vi "Dashboard Main.vi"() -> ()   [LabVIEW 2016]
uses:
  <vilib>/Utility/miscctls.llb/LVRowAndColumnTypeDef.ctl
  <vilib>/event_ctls.llb/eventvkey.ctl
  <vilib>/Rock Robotics/Network Tables/NT Read Numeric Array.vi
  <vilib>/Rock Robotics/Network Tables/NT Write Numeric Array.vi
  <vilib>/Rock Robotics/WPI/Dashboard/WPI_DashboardLogging Global.vi
panel:
  in  "Camera Settings Right":T1={"Frame Rate"=30, "Compression"=30, "Size"=1, "DB Camera Config"=FALSE} {"Frame Rate" scale=1.0..30.0; "Compression" scale=100.0..-1.0; "Size" items=["640x480", "320x240", "160x120"]}
  in  "Camera Name Right":string(combo)="No Camera Selection"
  out "Camera Info":cluster{"Mbps LED":bool, "Mbps":dbl, "fps":dbl} {"fps" format="%#.1g"; "Mbps" format="%#.1g"}
  in  "Camera Settings":T1={"Frame Rate"=30, "Compression"=30, "Size"=1, "DB Camera Config"=FALSE} {"Frame Rate" scale=1.0..30.0; "Compression" scale=100.0..-1.0; "Size" items=["640x480", "320x240", "160x120"]}
  in  "TCP":refnum<k5>
  in  "Rec Mode":enum32{"Stop", "Record", "Playback"}(radio)
  out "Robot IP":string
  out "Image Message":string="Timeout in Camera Communications"
  in  "Dashboard Tab":T2(tab)
  in  "Select Auto":string(combo)="Select Autonomous ..."
  out "NT Connection":bool
  out "MotorChart R":cluster{"Numeric":dbl, "Numeric":dbl}(graph)
  out "MotorChart L":cluster{"Numeric":dbl, "Numeric":dbl}(graph)
  out "MotorSliders R":cluster{"MotorSlide1":dbl, "MotorSlide2":dbl} {"MotorSlide2" scale=-1.0..1.0 scale format="%#_2e"; "MotorSlide1" scale=-1.0..1.0 scale format="%#_2e"}
  out "MotorSliders L":cluster{"MotorSlide1":dbl, "MotorSlide2":dbl} {"MotorSlide2" scale=-1.0..1.0 scale format="%#_2e"; "MotorSlide1" scale=-1.0..1.0 scale format="%#_2e"}
  out "Gyro":dbl(knob) scale=0.0..360.0
  out "JS1 Z":dbl(slide) scale=-1.0..1.0 scale format="%#_2e"
  out "JS1 Graph":cluster{"X":dbl, "Y":dbl}[](graph)
  out "JS1 Buttons":T3
  out "JS2 Z":dbl(slide) scale=-1.0..1.0 scale format="%#_2e"
  out "JS2 Graph":cluster{"X":dbl, "Y":dbl}[](graph)
  out "JS2 Buttons":T3
  out "Mode":T4(ring)=enum."Auto Disabled"
  out "Camera Image Right":T5(plugin-control)
  out "Left Encoder":dbl
  out "Right Encoder":dbl
  in  "Function Tuning":enum32{"Drive with PID", "Drive by Angle"}(tab)
  in  "Accel Distance":dbl=64.0
  in  "Min Speed":dbl=0.35
  in  "Drive P/I/D":dbl[](array[numeric])=[1.0, 0.0, 0.01]
  in  "Max Speed":dbl=0.6
  in  "Turn Speed":dbl=0.65
  in  "Linearity":dbl=0.6
  in  "Turn P/I/D":dbl[](array[numeric])=[0.25, 0.001, 0.0]
  in  "Autonomous Distances":T6(tab)
  in  "Station 1":dbl[](array[numeric])=[97.0, 30.0, -30.0, 120.0]
  in  "Station 2":dbl[](array[numeric])=[82.0, -48.0, 48.0, 120.0]
  in  "Station 3":dbl[](array[numeric])=[96.0, 30.0, -30.0, 120.0]
  in  "Drive Forward":dbl[](array[numeric])=[82.0, 0.0, 0.0, 0.0]
  in  "Gear and B":dbl[](array[numeric])=[82.0, -48.0, 0.0, 0.0]
  in  "Test Slider":dbl(slide) scale=0.0..100.0 scale format="%#_3g"
  in  "On/Off":bool caption="Solenoid"
  in  "Test Name":u16(ring) items=["Select the test to run..."]
  in  "Test Tree":string(tree)
  in  "Motor":cluster{"Value":dbl, "Enable":bool} {"Value" scale=-1.0..1.0 scale format="%#_3g"}
  out "Progress":T7 {"Test Progress" scale=0.0..100.0}
  in  "Rev/Fwd":cluster{"Forward":bool, "Reverse":bool}
  in  "Test Ring":u16(ring) items=["Monochrome", "Color"]
  out "Cmd Status":string
  in  "Execute Command":bool
  in  "Command Params":string[][](table)
  in  "Command Selection":i32(listbox)
  in  "CheckList":i32(listbox)
  out "Tree":string(tree)
  out "Camera Image":T5(plugin-control)
  in  "Camera Name":string(combo)="No Camera Selection"
  in  "Background":bool
  # "HW"
  # "HW"
  # "Joysticks"
  # "Drive Motors"
  # "Front"
  # "Right"
  # "Left"
  # "Back"
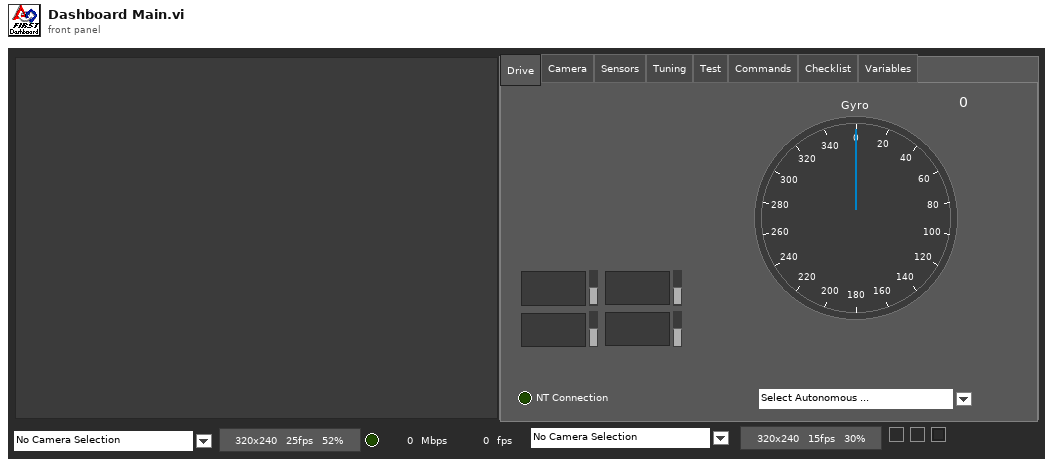
[diagram p1: front panel]
types:
  T1 = cluster{"Frame Rate":i32, "Compression":i32, "Size":u16, "DB Camera Config":bool}
  T2 = enum32{"Drive", "Camera", "Sensors", "Tuning", "Test", "Commands", "Checklist", "Variables"}
  T3 = cluster{bool, bool, bool, bool, bool, bool, bool, bool, bool, bool, bool, bool}
  T4 = enum8{"Tele-Op Disabled", "Tele-Op Enabled", "Auto Disabled", "Auto Enabled", "Test Disabled", "Test Enabled", "Disconnected", "No Code", "E-Stop"}
  T5 = typedef "IMAQ Image.ctl" = refnum<image>
  T6 = enum32{"Station 1", "Station 2", "Station 3", "Drive Forward", "Gear and Back"}
  T7 = cluster{"Test Progress":u8, "Test Progress Text":string}
  T8 = typedef "Image Type" = u32
  T9 = cluster{"IDs":cluster{"RPC field ID":u16, "Unique ID":u16}, "String":string}
  T10 = enum32{"Drive", "Basic", "Custom", "Test", "Checklist", "Variables"}
  T11 = cluster{"Error Strings":string, "Disable Counts":cluster{u16, u16}, "Rail Faults":cluster{u16, u16, u16}, "Robot IP":string, "DB Mode":u8, "Event Info":cluster{"Name":string, "Type":u8, "Number":u16, "Replay":u8}}
  T12 = cluster{"Storage":cluster{"Disk Free":u64, "RAM Block":u32, "RAM free":u32}, "CPU Utilization":cluster{"CPU % ISR":sgl, "CPU % Time Crit":sgl, "CPU % Timed Str":sgl, "CPU % High":sgl, "CPU % Above":sgl, "CPU % Normal":sgl, "CPU % Low":sgl}, "CAN":cluster{"% Bus Utilization":sgl, "Bus Off Cnt":u32, "TX_FIFO Full Cnt":u32, "Receive Error Cnt":u8, "Transmit Error Cnt":u8}, "HID":cluster{"HID Outputs":u32, "Rumble Low":u16, "Rumble High":u16}[]}
  T13 = cluster{"Status bits":cluster{"Test Mode":bool, "Autonomous":bool, "Enabled":bool, "Code Start":bool, "Brownout":bool, "Reserved 2":bool, "Reserved 3":bool, "E-Stop":bool}, "Code Trace":cluster{"Disabled":bool, "TeleOp":bool, "Auto":bool, "Test":bool}, "Controller Type":enum16{"unknown", "cRIO", "roboRio"}, "Code?":enum16{"unknown", "noCode", "code"}, "Battery V":dbl}
  T14 = cluster{"Control Bits":cluster{"TestMode":bool, "Autonomous":bool, "Enabled":bool, "FMS Present":bool, bool, bool, bool, "E-Stop":bool}, "Team Station ":u8, "Countdown":sgl, "Joystick Values":cluster{"Axes":dbl[], "Buttons":bool[], "POVs":i16[]}[]}
  T15 = cluster{"Axes":dbl[], "Buttons":bool[], "POVs":i16[]}[]
  T16 = cluster{"Axes":dbl[], "Buttons":bool[], "POVs":i16[]}
  T17 = cluster{"Buttons[0]":bool, "Buttons[1]":bool, "Buttons[2]":bool, "Buttons[3]":bool, "Buttons[4]":bool, "Buttons[5]":bool, "Buttons[6]":bool, "Buttons[7]":bool, "Buttons[8]":bool, "Buttons[9]":bool, "Buttons[10]":bool, "Buttons[11]":bool}
  T18 = cluster{"Camera Image":refnum<vi>, "Dashboard Tab":refnum<vi>, "Background":refnum<vi>, "Rec Mode":refnum<vi>, "Test Slider":refnum<vi>, "On/Off ":refnum<vi>, "Test Ring":refnum<vi>, "Rev/Fwd":refnum<vi>, "Test Name":refnum<vi>, "Motor":refnum<vi>, "Progress":refnum<vi>, "CheckList":refnum<vi>, "Tree":refnum<vi>, "Test Tree":refnum<vi>, "Command Params":refnum<vi>, "Command Selection":refnum<vi>, "Execute Command":refnum<vi>, "Cmd Status":refnum<vi>, "Camera Settings":refnum<vi>, "Camera Name":refnum<vi>, "Camera Info":refnum<vi>, "Camera Settings Right":refnum<vi>, "Camera Name Right":refnum<vi>, "Camera Image Right":refnum<vi>}
  T19 = cluster{"Operation":enum16{"Update", "Clear"}, "Color Box":u32}[]
  T20 = typedef "eventvkey.ctl" = enum16{"ASCII", "Enter", "Return", "Shift", "Ctrl", "Alt", "Cmd", "Opt", "Caps", "NumLock", "Clear", "Break", "Up", "Down", "Left", "Right", "Insert", "Delete", "Home", "End", "PageUp", "PageDown", "Escape", "Help", "Pause", "ScrollLock", "F1", "F2", "F3", "F4", "F5", "F6", "F7", "F8", "F9", "F10", "F11", "F12", "F13", "F14", "F15", "F16", "F17", "F18", "F19", "F20", "F21", "F22", "F23", "F24", "Play", "VolumeUp", "VolumeDown", "Mute", "Two Byte Char"}
  T21 = cluster{"Image Size":bool, "Image Type":bool, "Pixel Value":bool, "ROI Information":bool, "Zoom Factor":bool}
  T22 = cluster{"Operation":enum16{"Update", "Clear"}, "Color Box":u32}
  T23 = typedef "LVRowAndColumnTypeDef.ctl" = cluster{"Row":i32, "Column":i32}
  T24 = cluster{"Shift":bool, "Ctrl":bool, "Alt":bool, "Cmd":bool, "Opt":bool}
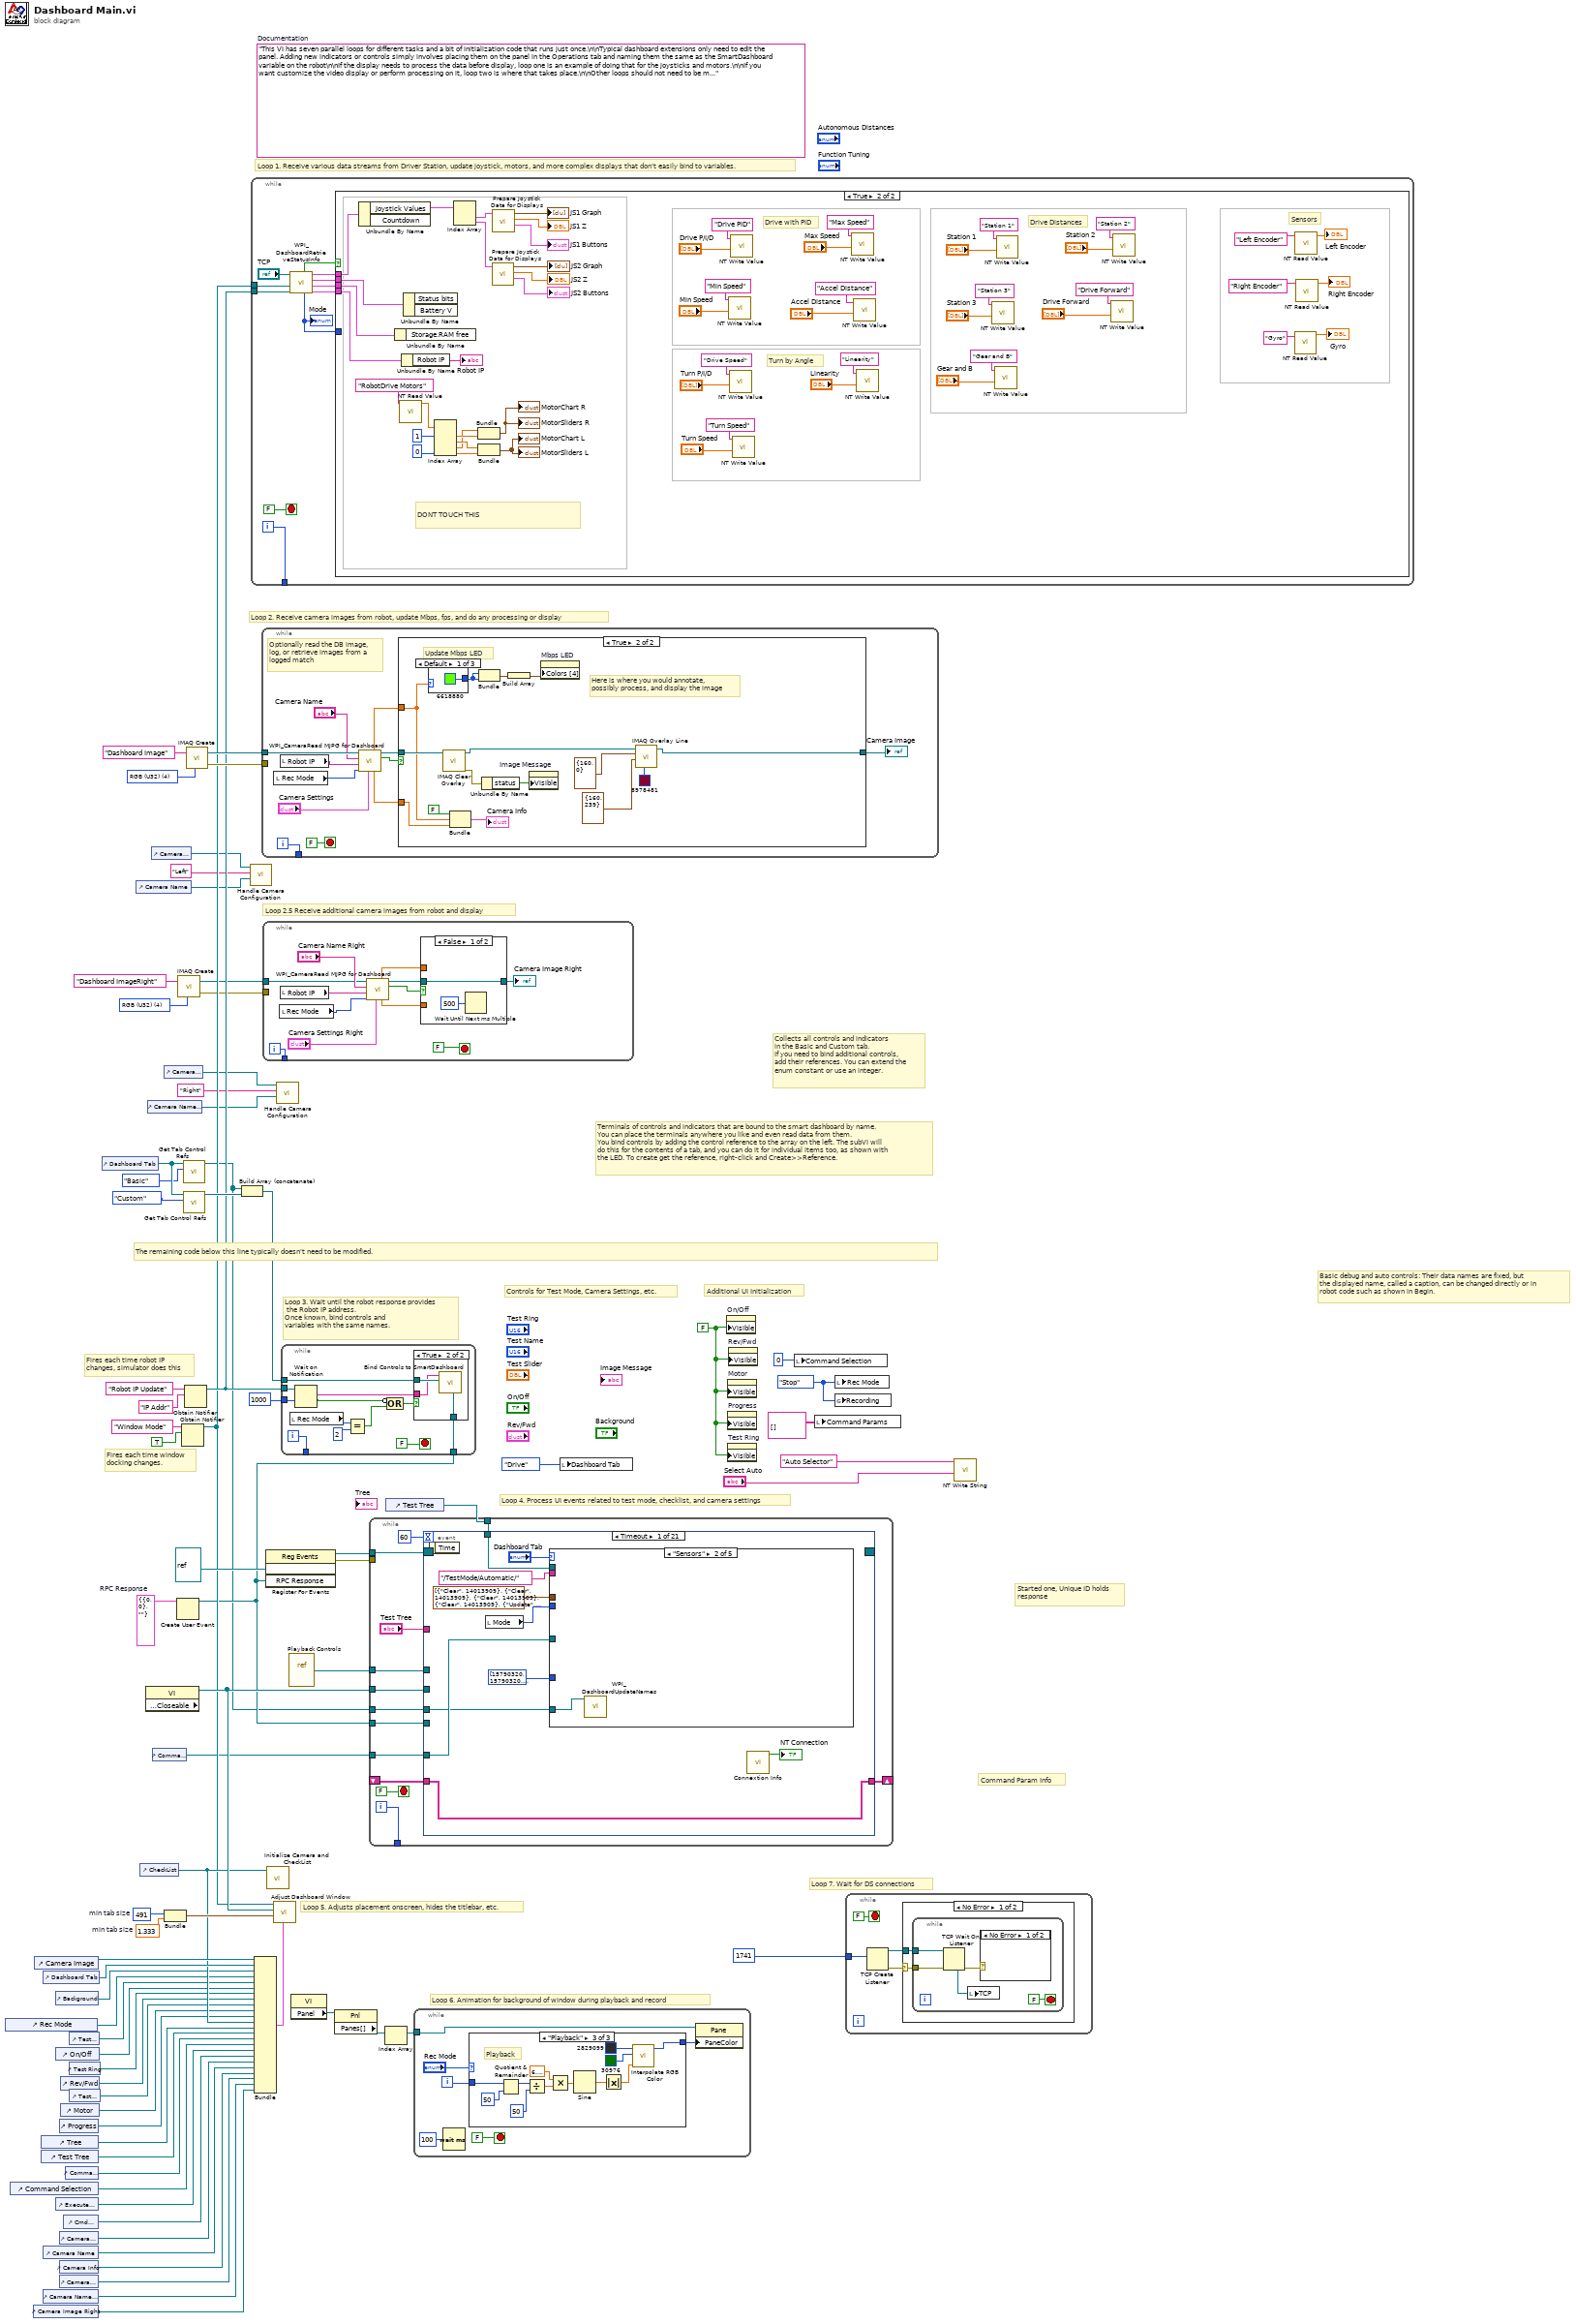
[diagram p0: block diagram]
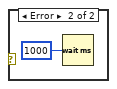
[diagram p3: hidden frame]
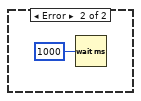
[diagram p4: hidden frame]
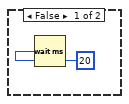
[diagram p5: hidden frame]
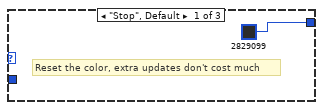
[diagram p6: hidden frame]
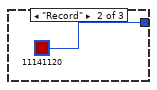
[diagram p7: hidden frame]
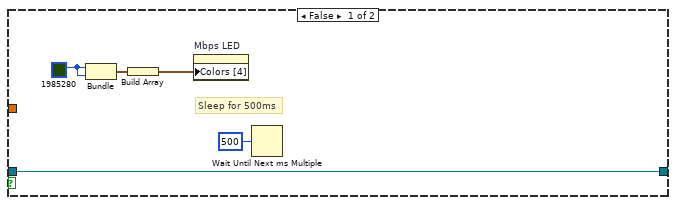
[diagram p9: hidden frame]
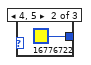
[diagram p10: hidden frame]
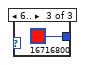
[diagram p11: hidden frame]
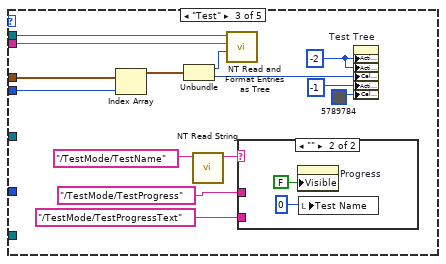
[diagram p13: hidden frame]
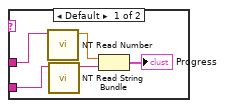
[diagram p14: hidden frame]
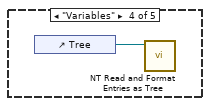
[diagram p15: hidden frame]
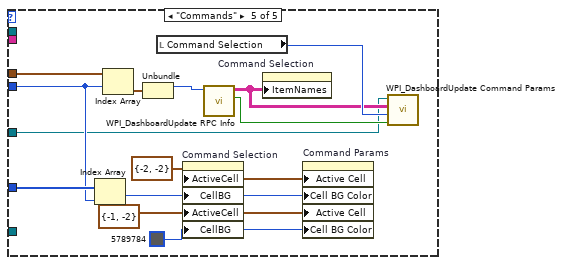
[diagram p16: hidden frame]
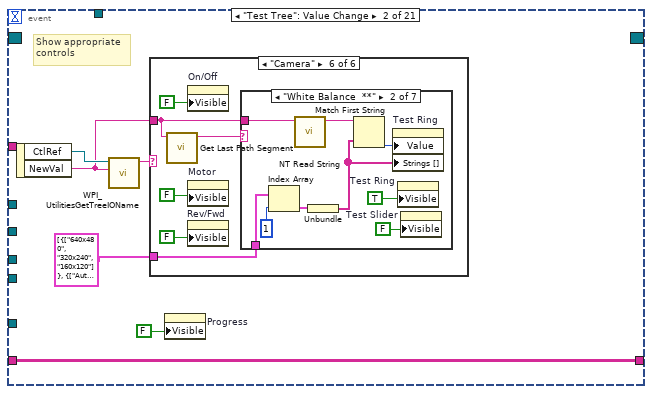
[diagram p17: hidden frame]
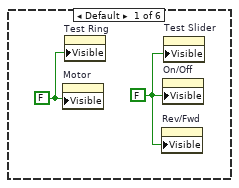
[diagram p18: hidden frame]
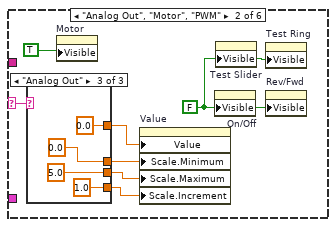
[diagram p19: hidden frame]
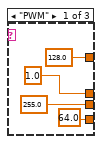
[diagram p20: hidden frame]
diagram:
  w11 = T8 4 items=["Grayscale (U8)", "Grayscale (I16)", "Grayscale (SGL)", "Complex (CSG)", "RGB (U32)", "HSL (U32)", "RGB (U64)"] ("Image Type")
  w27 = T9 {"IDs"={"RPC field ID"=0, "Unique ID"=0}, "String"=""}  # RPC Response
  w51 = 491  # min tab size
  w50 = 1.333  # min tab size
  w58 = enum32{"Stop", "Record", "Playback"}."Stop" ("Rec Mode")
  w34 = FALSE ("Visible")
  (unwired) "This VI has seven parallel loops for different tasks and a bit of initialization code that runs just once.\n\nTypical dashboard extensions only need to edit the panel. Adding new indicators or controls simply involves placing them on the panel in the Operations tab and naming them the same as the SmartDashboard variable on the robot\n\nIf the display needs to process the data before display, loop one is an example of doing that for the joysticks and motors.\n\nIf you want customize the video display or perform processing on it, loop two is where that takes place.\n\nOther loops should not need to be modified. They are pretty standard, and document the task they perform."  # Documentation
  w75 = T8 4 items=["Grayscale (U8)", "Grayscale (I16)", "Grayscale (SGL)", "Complex (CSG)", "RGB (U32)", "HSL (U32)", "RGB (U64)"] ("Image Type")
  # "Loop 2.5 Receive additional camera images from robot and display"
  # "Command Param Info"
  # "Started one, Unique ID holds\nresponse"
  # "Loop 7. Wait for DS connections"
  # "Basic debug and auto controls: Their data names are fixed, but\nthe displayed name, called a caption, can be changed directly or in\nrobot code such as shown in Begin."
  # "Controls for Test Mode, Camera Settings, etc."
  # "Additional UI Initialization"
  # "Loop 6. Animation for background of window during playback and record"
  # "Fires each time robot IP\nchanges, simulator does this"
  # "Fires each time window\ndocking changes."
  # "Collects all controls and indicators\nin the Basic and Custom tab.\nIf you need to bind additional controls,\nadd their references. You can extend the\nenum constant or use an integer."
  # "The remaining code below this line typically doesn't need to be modified."
  # "Loop 4. Process UI events related to test mode, checklist, and camera settings"
  # "Terminals of controls and indicators that are bound to the smart dashboard by name.\nYou can place the terminals anywhere you like and even read data from them.\nYou bind controls by adding the control reference to the array on the left. The subVI will\ndo this for the contents of a tab, and you can do it for individual items too, as shown with\nthe LED. To create get the reference, right-click and Create>>Reference."
  # "Loop 3. Wait until the robot response provides\n the Robot IP address.\nOnce known, bind controls and\nvariables with the same names."
  # "Loop 5. Adjusts placement onscreen, hides the titlebar, etc."
  # "Loop 1. Receive various data streams from Driver Station, update joystick, motors, and more complex displays that don't easily bind to variables."
  # "Loop 2. Receive camera images from robot, update Mbps, fps, and do any processing or display"
  n1 = control-ref of="Rec Mode"() -> (w40:refnum<vi>)
  n2 = control-ref of="Command Selection"() -> (w26:refnum<vi>)
  n3 = control-ref of="Camera Image Right"() -> (w2:refnum<vi>)
  n4 = control-ref of="Camera Image"() -> (w53:refnum<vi>)
  n5 = control-ref of="Tree"() -> (w44:refnum<vi>)
  n6 = control-ref of="Test Tree"() -> (w43:refnum<vi>)
  n7 = control-ref of="Dashboard Tab"() -> (w52:refnum<vi>)
  n8 = control-ref of="Camera Name"() -> (w17:refnum<vi>)
  n9 = control-ref of="Camera Name Right"() -> (w3:refnum<vi>)
  n10 = control-ref of="Background"() -> (w1:refnum<vi>)
  n11 = control-ref of="Execute Command"() -> (w28:refnum<vi>)
  n12 = control-ref of="On/Off"() -> (w38:refnum<vi>)
  n13 = control-ref of="Progress"() -> (w35:refnum<vi>)
  n14 = control-ref of="Camera Settings"() -> (w18:refnum<vi>)
  n15 = control-ref of="Camera Info"() -> (w16:refnum<vi>)
  n16 = control-ref of="Camera Settings Right"() -> (w4:refnum<vi>)
  n17 = control-ref of="Rev/Fwd"() -> (w36:refnum<vi>)
  n18 = control-ref of="Motor"() -> (w41:refnum<vi>)
  n19 = control-ref of="Cmd Status"() -> (w22:refnum<vi>)
  n20 = control-ref of="Command Params"() -> (w29:refnum<vi>)
  n21 = control-ref of="Test Slider"() -> (w39:refnum<vi>)
  n22 = control-ref of="Test Ring"() -> (w37:refnum<vi>)
  n23 = control-ref of="Test Name"() -> (w42:refnum<vi>)
  n24 = control-ref of="Dashboard Tab"() -> (w56:refnum<vi>)
  n25 = control-ref of="Camera Name"() -> (w19:refnum<vi>)
  n26 = control-ref of="CheckList"() -> (w45:refnum<vi>)
  n27 = property class="VI" props=["Front Panel.Closeable"]() -> (reference out=w57:refnum<vi>)  [unwired: 2 in, 2 out]
  n28 = control-ref of="Camera Name Right"() -> (w7:refnum<vi>)
  n29 = control-ref of="Camera Settings"() -> (w20:refnum<vi>)
  n30 = control-ref of="Command Params"() -> (w21:refnum<vi>)
  n31 = control-ref of="Camera Settings Right"() -> (w8:refnum<vi>)
  n32 = Bundle("min tab size"=w51, "min tab size"=w50) -> (w49:cluster{"min tab size":i32, "min tab size":dbl})  [unwired: 1 in]
  n33 = Create User Event(user event datatype=w27) -> (user event=w23:refnum<user-event>)  [unwired: 1 in, 1 out]
  n34 = call "IMAQ Create"("Image Name"="Dashboard ImageRight", "Image Type"=w11) -> ("New Image"=w10:T5, "error out"=w9:errorcluster)  [unwired: 2 in, 1 out]
  n35 = Obtain Notifier(name (unnamed)="Window Mode", notification data type=TRUE) -> (notifier out=w32:refnum<notifier>)  [unwired: 2 in, 2 out]
  n36 = call <vilib>:"Get Tab Control Refs.vi"("Page Index"=T10."Basic" ("Dashboard Tab"), "TabControl in"=w56) -> ("ControlsOnPage"=w15:refnum<vi>[])  [unwired: 9 in]
  n37 = call <vilib>:"Get Tab Control Refs.vi"("Page Index"=T10."Custom" ("Dashboard Tab"), "TabControl in"=w56) -> ("ControlsOnPage"=w55:refnum<vi>[])  [unwired: 9 in]
  n38 = Obtain Notifier(name (unnamed)="Robot IP Update", notification data type="IP Addr" ("name (unnamed)")) -> (notifier out=w33:refnum<notifier>)  [unwired: 2 in, 2 out]
  n39 = call "IMAQ Create"("Image Name"="Dashboard Image", "Image Type"=w75) -> ("New Image"=w73:T5, "error out"=w72:errorcluster)  [unwired: 2 in, 1 out]
  n40 = Build Array (concatenate)(w15, w55) -> (w54:refnum<vi>[])
  n41 = call "Handle Camera Configuration.vi"("CameraNameRef"=w19, "Camera File Name"="Left", "ClusterRef"=w20) -> ()  [unwired: 9 in]
  n42 = while {
    tunnel: [w85] -> _
    tunnel: w33 -> [w79]
    tunnel: w32 -> [w76]
    i -> [w85]
    stop <- FALSE stop-if-true
    n43 = call <vilib>:"WPI_DashboardRetrieveStatusInfo.vi"("Binding Refnum"=w79, "Window Mode Notifier"=w76, "TCP Cnx"="TCP") -> ("Power and Errors"=w80:T11, "Robot Metrics"=w83:T12, "Status Info"=w84:T13, "Control Info"=w81:T14, "Robot Mode"=w78:T4, "Process?"=w82:bool)  [unwired: 3 in]
    "Mode" <- w78
    n44 = case shown="True" w82 {
      tunnel: w84 -> [_ w141]
      tunnel: w83 -> [_ w140]
      tunnel: w81 -> [_ w139]
      tunnel: w80 -> [_ w138]
      tunnel: w78 -> [_ _]
      frame False {
        n45 = Wait (ms)(milliseconds to wait=u32 20) -> ()  [unwired: 1 out]
      }
      frame True {
        # "Sensors"
        # "Drive Distances"
        # "Turn by Angle"
        # "Drive with PID"
        # "DONT TOUCH THIS"
        n46 = Unbundle By Name(w139) -> ("Joystick Values"=w129:T15)  [unwired: 1 out]
        n47 = Unbundle By Name(w140) -> ()  [unwired: 1 out]
        n48 = call-poly <vilib>:"NT Read Value.vi"("Name"="RobotDrive Motors") -> ("Numeric Array"=w119:dbl[])  [unwired: 9 in, 1 out]
        n49 = Unbundle By Name(w138) -> ("Robot IP"=→"Robot IP":string)
        n50 = Unbundle By Name(w141) -> ()  [unwired: 2 out]
        n51 = Index Array(array=w119, index #1=1, index #4=0) -> (element #1=w133:dbl, element #2=w134:dbl, element #3=w132:dbl, element #4=w137:dbl)  [unwired: 2 in]
        n52 = Index Array(array=w129) -> (element #1=w128:T16, element #2=w124:T16)  [unwired: 2 in]
        n53 = Bundle("Numeric"=w132, "Numeric"=w133) -> (→"MotorChart R" →"MotorSliders R":cluster{"Numeric":dbl, "Numeric":dbl})  [unwired: 1 in]
        n54 = Bundle("Numeric"=w134, "Numeric"=w137) -> (→"MotorChart L" →"MotorSliders L":cluster{"Numeric":dbl, "Numeric":dbl})  [unwired: 1 in]
        n55 = call "Prepare Joystick Data for Displays.vi"("Joystick Values"=w124) -> ("Buttons"=→"JS2 Buttons":T17, "Z Axis"=→"JS2 Z":dbl, "Cartesian Data"=→"JS2 Graph":cluster{"X axis":dbl, "X axis":dbl}[])  [unwired: 8 in]
        n56 = call "Prepare Joystick Data for Displays.vi"("Joystick Values"=w128) -> ("Buttons"=→"JS1 Buttons":T17, "Z Axis"=→"JS1 Z":dbl, "Cartesian Data"=→"JS1 Graph":cluster{"X axis":dbl, "X axis":dbl}[])  [unwired: 8 in]
        n57 = call-poly <vilib>:"NT Write Value.vi"("Numeric"="Min Speed", "Name"="Min Speed") -> ()  [unwired: 9 in, 1 out]
        n58 = call-poly <vilib>:"NT Write Value.vi"("Numeric Array"="Turn P/I/D", "Name"="Drive Speed") -> ()  [unwired: 9 in, 1 out]
        n59 = call-poly <vilib>:"NT Write Value.vi"("Numeric Array"="Drive P/I/D", "Name"="Drive PID") -> ()  [unwired: 9 in, 1 out]
        n60 = call-poly <vilib>:"NT Write Value.vi"("Numeric"="Turn Speed", "Name"="Turn Speed") -> ()  [unwired: 9 in, 1 out]
        n61 = call-poly <vilib>:"NT Write Value.vi"("Numeric"="Max Speed", "Name"="Max Speed") -> ()  [unwired: 9 in, 1 out]
        n62 = call-poly <vilib>:"NT Write Value.vi"("Numeric"="Accel Distance", "Name"="Accel Distance") -> ()  [unwired: 9 in, 1 out]
        n63 = call-poly <vilib>:"NT Write Value.vi"("Numeric"="Linearity", "Name"="Linearity") -> ()  [unwired: 9 in, 1 out]
        n64 = call-poly <vilib>:"NT Write Value.vi"("Numeric Array"="Station 3", "Name"="Station 3") -> ()  [unwired: 9 in, 1 out]
        n65 = call-poly <vilib>:"NT Write Value.vi"("Numeric Array"="Gear and B", "Name"="Gear and B") -> ()  [unwired: 9 in, 1 out]
        n66 = call-poly <vilib>:"NT Write Value.vi"("Numeric Array"="Station 1", "Name"="Station 1") -> ()  [unwired: 9 in, 1 out]
        n67 = call-poly <vilib>:"NT Write Value.vi"("Numeric Array"="Drive Forward", "Name"="Drive Forward") -> ()  [unwired: 9 in, 1 out]
        n68 = call-poly <vilib>:"NT Write Value.vi"("Numeric Array"="Station 2", "Name"="Station 2") -> ()  [unwired: 9 in, 1 out]
        n69 = call-poly <vilib>:"NT Read Value.vi"("Name"="Gyro") -> ("Numeric"=→"Gyro":dbl)  [unwired: 9 in, 1 out]
        n70 = call-poly <vilib>:"NT Read Value.vi"("Name"="Left Encoder") -> ("Numeric"=→"Left Encoder":dbl)  [unwired: 9 in, 1 out]
        n71 = call-poly <vilib>:"NT Read Value.vi"("Name"="Right Encoder") -> ("Numeric"=→"Right Encoder":dbl)  [unwired: 9 in, 1 out]
      }
    }
  }
  n72 = Bundle("Camera Image"=w53, "Dashboard Tab"=w52, "Background"=w1, "Rec Mode"=w40, "Test Slider"=w39, "On/Off"=w38, "Test Ring"=w37, "Rev/Fwd"=w36, "Test Name"=w42, "Motor"=w41, "Progress"=w35, "CheckList"=w45, "Tree"=w44, "Test Tree"=w43, "Command Params"=w29, "Command Selection"=w26, "Execute Command"=w28, "Cmd Status"=w22, "Camera Settings"=w18, "Camera Name"=w17, "Camera Info"=w16, "Camera Settings Right"=w4, "Camera Name Right"=w3, "Camera Image Right"=w2) -> (w46:T18)  [unwired: 1 in]
  n73 = while {
    tunnel: w73 -> [w151]
    tunnel: w72 -> [_]
    tunnel: [w152] -> _
    i -> [w152]
    stop <- FALSE stop-if-true
    # "Optionally read the DB image,\nlog, or retrieve images from a\nlogged match"
    n74 = local read "Rec Mode"() -> (w147:enum32{"Stop", "Record", "Playback"})
    n75 = local read "Robot IP"() -> (w146:string)
    n76 = call <vilib>:"WPI_CameraRead MJPG for Dashboard.vi"("Camera Settings"="Camera Settings", "Rec Mode"=w147, "Robot IP"=w146, "Camera Name"="Camera Name", "Refnum in"=w151) -> ("Active"=w149:bool, "Refnum out"=w150:T5, "FPS"=w148:dbl, "Bandwidth (Mbps)"=w145:dbl)  [unwired: 3 in]
    n77 = case shown="True" w149 {
      tunnel: w150 -> [w154 w169]
      tunnel: w145 -> [_ w166]
      tunnel: w148 -> [_ w167]
      tunnel: [w154 w162] -> w142
      frame False {
        w156 = u32 1985280 ("Color Box")
        # "Sleep for 500ms"
        n78 = Bundle("Color Box"=w156, "Color Box"=w156) -> (w157:cluster{"Color Box":u32, "Color Box":u32})  [unwired: 1 out]
        n79 = Build Array(w157) -> (w155:cluster{"Color Box":u32, "Color Box":u32}[])
        n80 = property on="Mbps LED" class="Bool (strict)"("Colors [4]"=w155) -> ()  [unwired: 2 in, 2 out]
        n81 = Wait Until Next ms Multiple(millisecond multiple=u32 500) -> ()  [unwired: 1 out]
      }
      frame True {
        # "Here is where you would annotate,\npossibly process, and display the image"
        # "Update Mbps LED"
        n82 = case shown="Default" w166 {
          tunnel: [u32 6618880 ("Color Box") u32 16776722 ("Color Box") u32 16716800 ("Color Box")] -> w170
          frame Default {
          }
          frame 4, 5 {
          }
          frame 6.. {
          }
        }
        n83 = call "IMAQ Clear Overlay"("Image"=w169) -> ("error out"=w172:errorcluster, "Image Out"=w163:T5)  [unwired: 2 in, 7 out]
        n84 = Bundle(FALSE, "Bandwidth (Mbps)"=w166, "FPS"=w167) -> (→"Camera Info":cluster{bool, "Bandwidth (Mbps)":dbl, "FPS":dbl})  [unwired: 1 in]
        n85 = Bundle("Color Box"=w170, "Color Box"=w170) -> (w171:cluster{"Color Box":u32, "Color Box":u32})  [unwired: 1 out]
        n86 = Unbundle By Name(w172) -> ("status"=w173:bool)
        n87 = Build Array(w171) -> (w168:cluster{"Color Box":u32, "Color Box":u32}[])
        n88 = property on="Image Message" class="Str"("Visible"=w173) -> ()  [unwired: 2 in, 2 out]
        n89 = property on="Mbps LED" class="Bool (strict)"("Colors [4]"=w168) -> ()  [unwired: 2 in, 2 out]
        n90 = call "IMAQ Overlay Line"("Color"=u32 8978481, "End Point"=cluster{"X":i32, "Y":i32} {"X"=160, "Y"=239}, "Start Point"=cluster{"X":i32, "Y":i32} {"X"=160, "Y"=0}, "Image"=w163) -> ("Image Out"=w162:T5)  [unwired: 6 in, 1 out]
      }
    }
    "Camera Image" <- w142
  }
  n91 = while {
    tunnel: w10 -> [w187]
    tunnel: w9 -> [_]
    tunnel: [w181] -> _
    i -> [w181]
    stop <- FALSE stop-if-true
    n92 = local read "Rec Mode"() -> (w185:enum32{"Stop", "Record", "Playback"})
    n93 = local read "Robot IP"() -> (w186:string)
    n94 = call <vilib>:"WPI_CameraRead MJPG for Dashboard.vi"("Camera Settings"="Camera Settings Right", "Rec Mode"=w185, "Robot IP"=w186, "Camera Name"="Camera Name Right", "Refnum in"=w187) -> ("Active"=w180:bool, "Refnum out"=w183:T5, "FPS"=w178:dbl, "Bandwidth (Mbps)"=w179:dbl)  [unwired: 3 in]
    n95 = case shown="False" w180 {
      tunnel: w183 -> [w189 w191]
      tunnel: w179 -> [_ _]
      tunnel: w178 -> [_ _]
      tunnel: [w189 w191] -> w177
      frame False {
        n96 = Wait Until Next ms Multiple(millisecond multiple=u32 500) -> ()  [unwired: 1 out]
      }
      frame True {
      }
    }
    "Camera Image Right" <- w177
  }
  n97 = register-events(refnum<vi> refnum, w23) -> (reference out=w62:refnum<event-registration>, error out=w61:errorcluster)  [unwired: 2 in]
  n98 = call "Initialize Camera and CheckList.vi"("ListBox in"=w45) -> ()  [unwired: 11 in]
  n99 = call "Adjust Dashboard Window.vi"("Sizing Refnums"=w46, "Size Constraints"=w49, "VI"=w57, "WIn Mode"=w32) -> ()  [unwired: 8 in]
  n100 = call "Handle Camera Configuration.vi"("CameraNameRef"=w7, "Camera File Name"="Right", "ClusterRef"=w8) -> ()  [unwired: 9 in]
  n101 = while {
    tunnel: w54 -> [w203]
    tunnel: w33 -> [w201]
    tunnel: [w199] -> _
    tunnel: u32 1000 ("milliseconds to wait") -> [w198]
    tunnel: w23 -> [w192]
    i -> [w199]
    stop <- FALSE stop-if-true
    n102 = local read "Rec Mode"() -> (w194:enum32{"Stop", "Record", "Playback"})
    n103 = Wait on Notification(notifier=w201, timeout in ms (-1)=w198) -> (notification=w200:string, timed out?=w196:bool)  [unwired: 2 in, 2 out]
    n104 = Equal?(x=w194, y=u16 2 ("Rec Mode")) -> (x = y?=w195:bool)
    n105 = Compound Arithmetic op=OR(invert w196, w195) -> (w197:bool)
    n106 = case shown="True" w197 {
      tunnel: w203 -> [_ w206]
      tunnel: w200 -> [_ w205]
      tunnel: w192 -> [_ w204]
      frame False {
      }
      frame True {
        n107 = call <vilib>:"Bind Controls to SmartDashboard.vi"("RPC ref"=w204, "Bound Control Refs"=w206, "Server IP Address"=w205) -> ()  [unwired: 9 in]
      }
    }
  }
  n108 = vi-ref "Playback Controls.vi"() -> (w63:refnum<vi>)
  n109 = property class="VI"() -> ("Panel"=w65:refnum<vi>)  [unwired: 2 in, 2 out]
  n110 = property class="Pnl"(reference=w65) -> ("Panes[]"=w66:refnum<vi>[])  [unwired: 1 in, 2 out]
  n111 = Index Array(array=w66) -> (element=w64:refnum<vi>)  [unwired: 1 in]
  n112 = control-ref of="Test Tree"() -> (w67:refnum<vi>)
  n113 = while {
    tunnel: [w216] -> _
    tunnel: w67 -> [w215]
    tunnel: w63 -> [w214]
    tunnel: w62 -> [w213]
    tunnel: w61 -> [_]
    tunnel: w57 -> [w212]
    tunnel: w23 -> [w211]
    tunnel: w21 -> [w210]
    shift-right: [w209] -> _
    shift-left: _ -> [w208]
    tunnel: w15 -> [w207]
    i -> [w216]
    stop <- FALSE stop-if-true
    n114 = event shown="[0] Timeout" {
      selector: w213 -> [_ _ _ _ _ _ _ _ _ _ _ _ _ _ _ _ _ _ _ _ _]
      dyn-events: [_ _ _ _ _ _ _ _ _ _ _ _ _ _ _ _ w472 _ _ _ _] -> _
      timeout: u32 60 ("milliseconds to wait") -> [_ _ _ _ _ _ _ _ _ _ _ _ _ _ _ _ _ _ _ _ _]
      tunnel: w215 -> [w228 _ _ _ _ _ _ _ _ _ _ _ _ _ _ _ _ _ _ _ _]
      tunnel: "Test Tree" -> [_ _ _ _ _ _ _ _ _ _ _ w439 w447 w449 w453 w461 _ _ _ _ _]
      tunnel: w214 -> [_ _ _ _ _ _ _ _ _ _ _ _ _ _ _ _ w474 _ w492 _ _]
      tunnel: w212 -> [_ _ _ _ _ _ _ _ _ _ _ _ _ _ _ _ w470 _ _ _ _]
      tunnel: w211 -> [_ _ _ _ _ _ _ _ _ _ _ _ _ _ _ _ w466 _ _ _ _]
      tunnel: w210 -> [w223 _ _ _ _ _ w390 _ _ _ _ _ _ _ _ _ _ _ _ _ _]
      tunnel: [w222 w267 w369 w374 w383 w387 w388 w397 w407 w414 w426 w438 w445 w448 w452 w460 w465 w487 w489 w493 w504] -> w209
      tunnel: w208 -> [w222 w267 w369 w374 w383 w387 w388 _ _ w414 w426 w438 w445 w448 w452 w460 w465 w487 w489 w493 w504]
      tunnel: w207 -> [w220 _ _ _ _ _ _ _ _ _ _ _ _ _ _ _ _ _ _ _ _]
      event Timeout {
        n115 = event-data() -> ()  [unwired: 1 in, 1 out]
        n116 = local read "Mode"() -> (w225:T4)
        n117 = case shown="\"Sensors\"" "Dashboard Tab" {
          tunnel: w228 -> [_ _ w244 _ _]
          tunnel: "/TestMode/Automatic/" ("Name Pattern") -> [_ _ w243 _ _]
          tunnel: T19 [{"Operation"=enum."Clear", "Color Box"=14013909}, {"Operation"=enum."Clear", "Color Box"=14013909}, {"Operation"=enum."Clear", "Color Box"=14013909}, {"Operation"=enum."Clear", "Color Box"=14013909}, {"Operation"=enum."Update", "Color Box"=14013909}, {"Operation"=enum."Update", "Color Box"=16777215}, {"Operation"=enum."Clear", "Color Box"=14013909}, {"Operation"=enum."Clear", "Color Box"=14013909}, {"Operation"=enum."Clear", "Color Box"=14013909}] -> [_ _ w236 _ w260]
          tunnel: w225 -> [_ _ w235 _ w259]
          tunnel: u32[] [15790320, 15790320, 15790320, 15790320, 16777215, 16777215, 15790320, 15790320, 15790320] -> [_ _ _ _ w265]
          tunnel: w223 -> [_ _ _ _ w253]
          tunnel: w220 -> [_ w230 _ _ _]
          frame "Tuning", Default {
          }
          frame "Sensors" {
            n118 = call <vilib>:"WPI_DashboardUpdateNames.vi"("Controls on Tab"=w230) -> ()  [unwired: 11 in]
          }
          frame "Test" {
            w242 = -2 ("Active Item:Row Number")
            n119 = Index Array(array=w236, index=w235) -> (element=w237:T22)
            n120 = Unbundle(w237) -> ("Operation"=w238:enum16{"Update", "Clear"}, "Color Box"=w239:u32)
            n121 = call <vilib>:"NT Read String.vi"("Name"="/TestMode/TestName") -> ("String"=w233:string)  [unwired: 9 in, 1 out]
            n122 = call <vilib>:"NT Read and Format Entries as Tree.vi"("Operation"=w238, "Name Pattern"=w243, "Tree Refnum"=w244) -> ()  [unwired: 7 in, 2 out]
            n123 = case shown="\"\"" w233 {
              tunnel: "/TestMode/TestProgress" ("Name") -> [w246 _]
              tunnel: "/TestMode/TestProgressText" ("Name") -> [w245 _]
              frame Default {
                n124 = call <vilib>:"NT Read Number.vi"("Name"=w246) -> ("Numeric"=w247:dbl)  [unwired: 9 in, 1 out]
                n125 = call <vilib>:"NT Read String.vi"("Name"=w245) -> ("String"=w248:string)  [unwired: 9 in, 1 out]
                n126 = Bundle("Numeric"=w247, "String"=w248) -> (→"Progress":cluster{"Numeric":dbl, "String":string})  [unwired: 1 in]
              }
              frame "" {
                n127 = property on="Progress" class="Clust (strict)"("Visible"=FALSE) -> ()  [unwired: 2 in, 2 out]
                n128 = local write "Test Name"(u16 0) -> ()
              }
            }
            n129 = property on="Test Tree" class="Tree (strict)"("Active Item Row Number"=w242, "ActiveColNum"=w242, "CellBG"=w239, "Active Item Row Number"=-1 ("Active Item:Row Number"), "CellBG"=u32 5789784 ("Color Box")) -> ()  [unwired: 2 in, 2 out]
          }
          frame "Variables" {
            n130 = control-ref of="Tree"() -> (w252:refnum<vi>)
            n131 = call <vilib>:"NT Read and Format Entries as Tree.vi"("Tree Refnum"=w252) -> ()  [unwired: 9 in, 2 out]
          }
          frame "Commands" {
            w261 = u32 5789784 ("Color Box")
            w262 = T23 {"Row"=-1, "Column"=-2} ("Active Cell:Active Cell")
            w264 = T23 {"Row"=-2, "Column"=-2} ("Active Cell:Active Cell")
            n132 = Index Array(array=w265, index=w259) -> (element=w263:u32)
            n133 = Index Array(array=w260, index=w259) -> (element=w258:T22)
            n134 = Unbundle(w258) -> ("Operation"=w257:enum16{"Update", "Clear"})  [unwired: 1 out]
            n135 = local read "Command Selection"() -> (w256:i32)
            n136 = property on="Command Selection" class="MCListbox (strict)"("ActiveCell"=w264, "CellBG"=w263, "ActiveCell"=w262, "CellBG"=w261) -> ()  [unwired: 2 in, 2 out]
            n137 = call <vilib>:"WPI_DashboardUpdate RPC Info.vi"("Operation"=w257) -> ("update"=w255:bool, "commands"=w254:string[][])  [unwired: 9 in]
            n138 = property on="Command Selection" class="MCListbox (strict)"("ItemNames"=w254) -> ()  [unwired: 2 in, 2 out]
            n139 = property on="Command Params" class="Tbl (strict)"("Active Cell"=w264, "Cell BG Color"=w263, "Active Cell"=w262, "Cell BG Color"=w261) -> ()  [unwired: 2 in, 2 out]
            n140 = call <vilib>:"WPI_DashboardUpdate Command Params.vi"("Update"=w255, "NewVal"=w256, "Commands"=w254, "Param Tbl"=w253) -> ()  [unwired: 7 in, 1 out]
          }
        }
        n141 = call <vilib>:"Connextion Info.vi"() -> ("Connected"=→"NT Connection":bool)  [unwired: 10 in, 1 out]
      }
      event "Test Tree": Value Change {
        # "Show appropriate\ncontrols"
        n142 = event-data() -> ("CtlRef"=w270:refnum<vi>, "NewVal"=w268:string)  [unwired: 1 in]
        n143 = call <vilib>:"WPI_UtilitiesGetTreeIOName.vi"("NewVal"=w268, "TreeControl in"=w270) -> ("I/O Name"=w271:string)  [unwired: 9 in]
        n144 = case shown="\"Camera\"" w271 {
          selector: w271 -> [_ w278 _ w300 w309 _]
          tunnel: w268 -> [_ _ w297 w299 _ w316]
          tunnel: cluster{string[]}[] [{["640x480", "320x240", "160x120"]}, {["Auto", "Fixed indoor", "Fixed outdoor 1", "Fixed outdoor 2", "Fixed fluorescent 1", "Fixed fluorescent 2", "Hold current"]}, {["Auto", "Flicker-free 50 Hz", "Flicker-free 60 Hz", "Hold current"]}, {["None", "Prioritize frame rate", "Prioritize image quality"]}, {["Monochrome", "Color"]}] -> [_ _ _ _ _ w315]
          frame Default {
            w273 = FALSE ("Visible")
            w272 = FALSE ("Visible")
            n145 = property on="Motor" class="Clust (strict)"("Visible"=w272) -> ()  [unwired: 2 in, 2 out]
            n146 = property on="Test Ring" class="Ring (strict)"("Visible"=w272) -> ()  [unwired: 2 in, 2 out]
            n147 = property on="Rev/Fwd" class="Clust (strict)"("Visible"=w273) -> ()  [unwired: 2 in, 2 out]
            n148 = property on="On/Off" class="Bool (strict)"("Visible"=w273) -> ()  [unwired: 2 in, 2 out]
            n149 = property on="Test Slider" class="Slide (strict)"("Visible"=w273) -> ()  [unwired: 2 in, 2 out]
          }
          frame "Analog Out", "Motor", "PWM" {
            w279 = FALSE ("Visible")
            n150 = case shown="\"Analog Out\"" w278 {
              tunnel: [1.0 ("Value") -1.0 ("Value") 0.0 ("Value")] -> w277
              tunnel: [255.0 ("Value") 1.0 ("Value") 5.0 ("Value")] -> w276
              tunnel: [128.0 ("Value") 0.0 ("Value") 0.0 ("Value")] -> w275
              tunnel: [64.0 ("Value") 0.5 ("Value") 1.0 ("Value")] -> w274
              frame "PWM" {
              }
              frame "Motor", Default {
              }
              frame "Analog Out" {
              }
            }
            n151 = property on="Motor" class="Clust (strict)"("Visible"=TRUE) -> ()  [unwired: 2 in, 2 out]
            n152 = property on="Value" class="Slide (strict)"("Value"=w275, "Scale.Minimum"=w277, "Scale.Maximum"=w276, "Scale.Increment"=w274) -> ()  [unwired: 2 in, 2 out]
            n153 = property on="On/Off" class="Bool (strict)"("Visible"=w279) -> ()  [unwired: 2 in, 2 out]
            n154 = property on="Test Slider" class="Slide (strict)"("Visible"=w279) -> ()  [unwired: 2 in, 2 out]
            n155 = property on="Test Ring" class="Ring (strict)"("Visible"=w279) -> ()  [unwired: 2 in, 2 out]
            n156 = property on="Rev/Fwd" class="Clust (strict)"("Visible"=w279) -> ()  [unwired: 2 in, 2 out]
          }
          frame "Servo" {
            w295 = FALSE ("Visible")
            n157 = call <vilib>:"NT Read Number.vi"("Name"=w297) -> ("Numeric"=w296:dbl)  [unwired: 9 in, 1 out]
            n158 = property on="Test Slider" class="Slide (strict)"("Visible"=TRUE, "Scale.Maximum"=170.0 ("Scale.Range:Maximum")) -> ()  [unwired: 2 in, 2 out]
            n159 = local write "Test Slider"(w296) -> ()
            n160 = property on="Motor" class="Clust (strict)"("Visible"=w295) -> ()  [unwired: 2 in, 2 out]
            n161 = property on="Rev/Fwd" class="Clust (strict)"("Visible"=w295) -> ()  [unwired: 2 in, 2 out]
            n162 = property on="On/Off" class="Bool (strict)"("Visible"=w295) -> ()  [unwired: 2 in, 2 out]
            n163 = property on="Test Ring" class="Ring (strict)"("Visible"=w295) -> ()  [unwired: 2 in, 2 out]
          }
          frame "Relay", "Solenoid" {
            w298 = FALSE ("Visible")
            n164 = property on="Motor" class="Clust (strict)"("Visible"=w298) -> ()  [unwired: 2 in, 2 out]
            n165 = property on="Test Slider" class="Slide (strict)"("Visible"=w298) -> ()  [unwired: 2 in, 2 out]
            n166 = Search and Replace String(input string=w299, search string="/Value  **", replace string="/Direction") -> (result string=w305:string)  [unwired: 5 in, 3 out]
            n167 = property on="Test Ring" class="Ring (strict)"("Visible"=w298) -> ()  [unwired: 2 in, 2 out]
            n168 = call <vilib>:"NT Read String.vi"("Name"=w305) -> ("String"=w303:string)  [unwired: 9 in, 1 out]
            n169 = Equal?(x="Both directions", y=w303) -> (x = y?=w301:bool)
            n170 = Not(x=w301) -> (.not. x?=w302:bool)
            n171 = property on="Rev/Fwd" class="Clust (strict)"("Visible"=w301) -> ()  [unwired: 2 in, 2 out]
            n172 = property on="On/Off" class="Bool (strict)"("Visible"=w302, "Caption.Text"=w300) -> ()  [unwired: 2 in, 2 out]
          }
          frame "Compressor", "Digital Out" {
            w308 = FALSE ("Visible")
            # "Get direction and finish"
            n173 = property on="Motor" class="Clust (strict)"("Visible"=w308) -> ()  [unwired: 2 in, 2 out]
            n174 = property on="Test Slider" class="Slide (strict)"("Visible"=w308) -> ()  [unwired: 2 in, 2 out]
            n175 = property on="Test Ring" class="Ring (strict)"("Visible"=w308) -> ()  [unwired: 2 in, 2 out]
            n176 = property on="On/Off" class="Bool (strict)"("Visible"=TRUE, "Caption.Text"=w309) -> ()  [unwired: 2 in, 2 out]
            n177 = property on="Rev/Fwd" class="Clust (strict)"("Visible"=FALSE) -> ()  [unwired: 2 in, 2 out]
          }
          frame "Camera" {
            n178 = call <vilib>:"Get Last Path Segment.vi"("String in"=w316) -> ("String out"=w317:string)  [unwired: 10 in]
            n179 = property on="On/Off" class="Bool (strict)"("Visible"=FALSE) -> ()  [unwired: 2 in, 2 out]
            n180 = property on="Motor" class="Clust (strict)"("Visible"=FALSE) -> ()  [unwired: 2 in, 2 out]
            n181 = property on="Rev/Fwd" class="Clust (strict)"("Visible"=FALSE) -> ()  [unwired: 2 in, 2 out]
            n182 = case shown="\"White Balance  **\"" w317 {
              tunnel: w316 -> [w323 w332 w341 w350 w359 _ w365]
              tunnel: w315 -> [w321 w329 w338 w347 w356 _ _]
              frame "Size  **" {
                n183 = Index Array(array=w321) -> (element=w320:cluster{string[]})  [unwired: 1 in]
                n184 = call <vilib>:"NT Read String.vi"("Name"=w323) -> ("String"=w322:string)  [unwired: 9 in, 1 out]
                n185 = Unbundle(w320) -> (w318:string[])
                n186 = Match First String(2:w318, 3:w322) -> (0:w319:i32)  [unwired: 1 out]
                n187 = property on="Test Ring" class="Ring (strict)"("Value"=w319, "Strings []"=w318) -> ()  [unwired: 2 in, 2 out]
                n188 = property on="Test Ring" class="Ring (strict)"("Visible"=TRUE) -> ()  [unwired: 2 in, 2 out]
                n189 = property on="Test Slider" class="Slide (strict)"("Visible"=FALSE) -> ()  [unwired: 2 in, 2 out]
              }
              frame "White Balance  **" {
                n190 = Index Array(array=w329, index=1) -> (element=w330:cluster{string[]})
                n191 = call <vilib>:"NT Read String.vi"("Name"=w332) -> ("String"=w331:string)  [unwired: 9 in, 1 out]
                n192 = Unbundle(w330) -> (w327:string[])
                n193 = Match First String(2:w327, 3:w331) -> (0:w326:i32)  [unwired: 1 out]
                n194 = property on="Test Ring" class="Ring (strict)"("Value"=w326, "Strings []"=w327) -> ()  [unwired: 2 in, 2 out]
                n195 = property on="Test Ring" class="Ring (strict)"("Visible"=TRUE) -> ()  [unwired: 2 in, 2 out]
                n196 = property on="Test Slider" class="Slide (strict)"("Visible"=FALSE) -> ()  [unwired: 2 in, 2 out]
              }
              frame "Exposure  **" {
                n197 = Index Array(array=w338, index=2) -> (element=w339:cluster{string[]})
                n198 = call <vilib>:"NT Read String.vi"("Name"=w341) -> ("String"=w340:string)  [unwired: 9 in, 1 out]
                n199 = Unbundle(w339) -> (w335:string[])
                n200 = Match First String(2:w335, 3:w340) -> (0:w336:i32)  [unwired: 1 out]
                n201 = property on="Test Ring" class="Ring (strict)"("Value"=w336, "Strings []"=w335) -> ()  [unwired: 2 in, 2 out]
                n202 = property on="Test Ring" class="Ring (strict)"("Visible"=TRUE) -> ()  [unwired: 2 in, 2 out]
                n203 = property on="Test Slider" class="Slide (strict)"("Visible"=FALSE) -> ()  [unwired: 2 in, 2 out]
              }
              frame "Exposure Priority  **" {
                n204 = Index Array(array=w347, index=3) -> (element=w348:cluster{string[]})
                n205 = call <vilib>:"NT Read String.vi"("Name"=w350) -> ("String"=w349:string)  [unwired: 9 in, 1 out]
                n206 = Unbundle(w348) -> (w344:string[])
                n207 = Match First String(2:w344, 3:w349) -> (0:w345:i32)  [unwired: 1 out]
                n208 = property on="Test Ring" class="Ring (strict)"("Value"=w345, "Strings []"=w344) -> ()  [unwired: 2 in, 2 out]
                n209 = property on="Test Ring" class="Ring (strict)"("Visible"=TRUE) -> ()  [unwired: 2 in, 2 out]
                n210 = property on="Test Slider" class="Slide (strict)"("Visible"=FALSE) -> ()  [unwired: 2 in, 2 out]
              }
              frame "Color Enable  **" {
                n211 = Index Array(array=w356, index=4) -> (element=w357:cluster{string[]})
                n212 = call <vilib>:"NT Read String.vi"("Name"=w359) -> ("String"=w358:string)  [unwired: 9 in, 1 out]
                n213 = Unbundle(w357) -> (w353:string[])
                n214 = Match First String(2:w353, 3:w358) -> (0:w354:i32)  [unwired: 1 out]
                n215 = property on="Test Ring" class="Ring (strict)"("Value"=w354, "Strings []"=w353) -> ()  [unwired: 2 in, 2 out]
                n216 = property on="Test Ring" class="Ring (strict)"("Visible"=TRUE) -> ()  [unwired: 2 in, 2 out]
                n217 = property on="Test Slider" class="Slide (strict)"("Visible"=FALSE) -> ()  [unwired: 2 in, 2 out]
              }
              frame Default {
                n218 = property on="Test Ring" class="Ring (strict)"("Visible"=FALSE) -> ()  [unwired: 2 in, 2 out]
                n219 = property on="Test Slider" class="Slide (strict)"("Visible"=FALSE) -> ()  [unwired: 2 in, 2 out]
              }
              frame "Brightness  **", "Color Level  **", "Compression  **", "FPS  **", "Sharpness  **" {
                n220 = call <vilib>:"NT Read Number.vi"("Name"=w365) -> ("Numeric"=w364:dbl)  [unwired: 9 in, 1 out]
                n221 = local write "Test Slider"(w364) -> ()
                n222 = property on="Test Slider" class="Slide (strict)"("Visible"=TRUE, "Scale.Maximum"=100.0 ("Scale.Range:Maximum")) -> ()  [unwired: 2 in, 2 out]
                n223 = property on="Test Ring" class="Ring (strict)"("Visible"=FALSE) -> ()  [unwired: 2 in, 2 out]
              }
            }
          }
        }
        n224 = property on="Progress" class="Clust (strict)"("Visible"=FALSE) -> ()  [unwired: 2 in, 2 out]
      }
      event "Test Name": Mouse Enter {
        # "Populate the ring with the list of tests"
        n225 = event-data() -> ()  [unwired: 1 in, 1 out]
        n226 = call <vilib>:"NT Read String Array.vi"("Name"="/TestMode/TestList") -> ("String Array"=w373:string[])  [unwired: 9 in, 1 out]
        n227 = Build Array (concatenate)("Select the test to run...", w373) -> (w372:string[])
        n228 = property on="Test Name" class="Ring (strict)"("Strings []"=w372) -> ()  [unwired: 2 in, 2 out]
      }
      event "Test Name": Value Change {
        w375 = FALSE ("Visible")
        # "Tell the robot the test name to run"
        n229 = event-data() -> ("NewVal"=w379:u16)  [unwired: 1 in]
        n230 = property on="Test Name" class="Ring (strict)"() -> ("Strings []"=w380:string[])  [unwired: 2 in, 2 out]
        n231 = local write "Progress"(T7 {"Test Progress"=0, "Test Progress Text"=""} ("Progress")) -> ()
        n232 = Index Array(array=w380, index=w379) -> (element=w378:string)
        n233 = call <vilib>:"NT Write String.vi"("String"=w378, "Name"="/TestMode/TestName") -> ()  [unwired: 9 in, 1 out]
        n234 = property on="Progress" class="Clust (strict)"("Visible"=TRUE) -> ()  [unwired: 2 in, 2 out]
        n235 = property on="Motor" class="Clust (strict)"("Visible"=w375) -> ()  [unwired: 2 in, 2 out]
        n236 = property on="Test Slider" class="Slide (strict)"("Visible"=w375) -> ()  [unwired: 2 in, 2 out]
        n237 = property on="On/Off" class="Bool (strict)"("Visible"=w375) -> ()  [unwired: 2 in, 2 out]
        n238 = property on="Rev/Fwd" class="Clust (strict)"("Visible"=w375) -> ()  [unwired: 2 in, 2 out]
        n239 = property on="Test Ring" class="Ring (strict)"("Visible"=w375) -> ()  [unwired: 2 in, 2 out]
      }
      event "Select Auto": Mouse Enter {
        # "Populate the combo box with the list of autonomous options"
        n240 = event-data() -> ()  [unwired: 1 in, 1 out]
        n241 = call <vilib>:"NT Read String Array.vi"("Name"="Auto List") -> ("String Array"=w382:string[])  [unwired: 9 in, 1 out]
        n242 = property on="Select Auto" class="CmbBox"("Strings[]"=w382) -> ()  [unwired: 2 in, 2 out]
      }
      event "Select Auto": Value Change {
        # "User modified the Auto Selection. Write to NT variable so robot knows."
        n243 = event-data() -> ("NewVal"=w385:string)  [unwired: 1 in]
        n244 = call <vilib>:"NT Write String.vi"("String"=w385, "Name"="Auto Selector") -> ()  [unwired: 9 in, 1 out]
      }
      event "Command Selection": Value Change {
        # "Get the params and show in table"
        n245 = event-data() -> ("NewVal"=w391:i32)  [unwired: 1 in]
        n246 = property on="Command Selection" class="MCListbox (strict)"() -> ("ItemNames"=w389:string[][])  [unwired: 2 in, 2 out]
        n247 = call <vilib>:"WPI_DashboardUpdate Command Params.vi"("NewVal"=w391, "Commands"=w389, "Param Tbl"=w390) -> ()  [unwired: 8 in, 1 out]
      }
      event "Execute Command": Value Change {
        # "Started one, Unique ID holds\nresponse"
        n248 = event-data() -> ()  [unwired: 1 in, 1 out]
        n249 = property on="Command Selection" class="MCListbox (strict)"() -> ("ItemNames"=w402:string[][])  [unwired: 2 in, 2 out]
        n250 = Index Array(array=w402, index (row)="Command Selection", index (col)=0) -> (element=w400:string)
        n251 = call <vilib>:"Invoke Commands.vi"("Command Params"="Command Params", "Function Name"=w400) -> ("Params"=w396:u8, "Started"=w395:bool)  [unwired: 7 in, 1 out]
        n252 = Array Subset(array="Command Params", length (row)=w396) -> (w397:string[][])  [unwired: 3 in]
        n253 = Select(t="Executing" ("Cmd Status"), s=w395, f="" ("Cmd Status")) -> (s? t:f=→"Cmd Status":string)
      }
      event "Command Selection": Double Click {
        n254 = event-data() -> ("Row"=w410:i32)  [unwired: 1 in]
        n255 = property on="Command Selection" class="MCListbox (strict)"() -> ("ItemNames"=w413:string[][])  [unwired: 2 in, 2 out]
        n256 = local read "Command Params"() -> (w409:string[][])
        n257 = Index Array(array=w413, index (row)=w410, index (col)=0) -> (element=w411:string)
        n258 = call <vilib>:"Invoke Commands.vi"("Command Params"=w409, "Function Name"=w411) -> ("Params"=w408:u8, "Started"=w403:bool)  [unwired: 7 in, 1 out]
        n259 = Array Subset(array=w409, length (row)=w408) -> (w407:string[][])  [unwired: 3 in]
        n260 = Select(t="Executing" ("Cmd Status"), s=w403, f="" ("Cmd Status")) -> (s? t:f=w404:string)
        n261 = local write "Cmd Status"(w404) -> ()
      }
      event "CheckList": Double Click {
        # "Shift clears all"
        # "Update symbols on the listbox"
        n262 = event-data() -> ("PlatMods.Shift"=w415:bool, "Row"=w417:i32)  [unwired: 1 in]
        n263 = case shown="True" w415 {
          tunnel: w417 -> [w421 _]
          tunnel: 1 -> [w420 _]
          frame False {
            n264 = property on="CheckList" class="LstBox (strict)"() -> ("Item Symbols"=w419:i32[])  [unwired: 2 in, 2 out]
            n265 = Replace Array Subset(array=w419, new element=w420, index=w421) -> (w418:i32[])
            n266 = property on="CheckList" class="LstBox (strict)"("Item Symbols"=w418) -> ()  [unwired: 2 in, 2 out]
          }
          frame True {
            w422 = 0 ("Top Row")
            n267 = property on="CheckList" class="LstBox (strict)"() -> ("Number of Rows"=w424:u32)  [unwired: 2 in, 2 out]
            n268 = Initialize Array(0, w424) -> (w423:i32[])
            n269 = property on="CheckList" class="LstBox (strict)"("Top Row"=w422, "Value"=w422, "Item Symbols"=w423) -> ()  [unwired: 2 in, 2 out]
          }
        }
      }
      event "CheckList": Key Down {
        # "Update symbols on the listbox\nLeft and right keys check and uncheck"
        n270 = event-data() -> ("VKey"=w428:T20)  [unwired: 1 in]
        n271 = case shown="\"Left\", \"Right\"" w428 {
          selector: w428 -> [w433 _]
          tunnel: eventvkey."Left" ("VKey") -> [w431 _]
          frame "Left", "Right" {
            n272 = Equal?(x=w431, y=w433) -> (x = y?=w432:bool)
            n273 = Select(t=0, s=w432, f=1) -> (s? t:f=w434:i32)
            n274 = property on="CheckList" class="LstBox (strict)"() -> ("Item Symbols"=w437:i32[])  [unwired: 2 in, 2 out]
            n275 = Replace Array Subset(array=w437, new element=w434, index="CheckList") -> (w436:i32[])
            n276 = property on="CheckList" class="LstBox (strict)"("Item Symbols"=w436) -> ()  [unwired: 2 in, 2 out]
          }
          frame Default {
          }
        }
      }
      event "Motor.Enable": Value Change {
        # "When the test mode otor enable helper is set, update that\ntree row item's value"
        n277 = event-data() -> ("NewVal"=w443:bool)  [unwired: 1 in]
        n278 = Unbundle("Motor") -> ("Value"=w442:dbl)  [unwired: 1 out]
        n279 = Select(t=w442, s=w443, f=0.0) -> (s? t:f=w440:dbl)
        n280 = call <vilib>:"NT Write Number.vi"("Numeric"=w440, "Name"=w439) -> ()  [unwired: 9 in, 1 out]
      }
      event "Test Slider": Value Change {
        # "When the test mode slider helper is set, update that\ntree row item's value"
        n281 = event-data() -> ("NewVal"=w446:dbl)  [unwired: 1 in]
        n282 = call <vilib>:"NT Write Number.vi"("Numeric"=w446, "Name"=w447) -> ()  [unwired: 9 in, 1 out]
      }
      event "On/Off": Value Change {
        # "When the test mode on/off helper value is set, update that\ntree row item's value"
        n283 = event-data() -> ("NewVal"=w451:bool)  [unwired: 1 in]
        n284 = Boolean To (0,1)(Boolean=w451) -> (0, 1=w450:i16)
        n285 = call <vilib>:"NT Write Number.vi"("Numeric"=w450, "Name"=w449) -> ()  [unwired: 9 in, 1 out]
      }
      event "Rev/Fwd": Value Change {
        # "When the test mode helper value for relays is set, update that\ntree row item's value"
        n286 = event-data() -> ("NewVal.Forward"=w459:bool, "NewVal.Reverse"=w458:bool)  [unwired: 1 in]
        n287 = Boolean To (0,1)(Boolean=w459) -> (0, 1=w455:i16)
        n288 = Boolean To (0,1)(Boolean=w458) -> (0, 1=w457:i16)
        n289 = Negate(x=w457) -> (-x=w456:i16)
        n290 = Add(x=w455, y=w456) -> (x+y=w454:i16)
        n291 = call <vilib>:"NT Write Number.vi"("Numeric"=w454, "Name"=w453) -> ()  [unwired: 9 in, 1 out]
      }
      event "Test Ring": Value Change {
        # "When a test mode helper value is selected from the ring,\nset the tree item's variable to the string value"
        n292 = event-data() -> ("NewVal"=w463:u16)  [unwired: 1 in]
        n293 = property on="Test Ring" class="Ring (strict)"() -> ("Strings []"=w464:string[])  [unwired: 2 in, 2 out]
        n294 = Index Array(array=w464, index=w463) -> (element=w462:string)
        n295 = call <vilib>:"NT Write String.vi"("String"=w462, "Name"=w461) -> ()  [unwired: 9 in, 1 out]
      }
      event "Rec Mode": Value Change {
        # "Update globals for recording mode and path to read log from.\nClear when logging and let NetworkTables set path for vision to\nuse."
        n296 = event-data() -> ("NewVal"=w475:enum32{"Stop", "Record", "Playback"})  [unwired: 1 in]
        n297 = global write "WPI_DashboardLogging Global.vi" "Logging Filename"(path "") -> ()
        n298 = global write "WPI_DashboardLogging Global.vi" "Recording"(w475) -> ()
        n299 = case shown="\"Playback\"" w475 {
          tunnel: w474 -> [_ w477 w486]
          tunnel: [_ _ w485] -> w472
          tunnel: [_ _ w484] -> _
          tunnel: w470 -> [_ _ w482]
          tunnel: cluster{i32, i32} {-250, 170} -> [_ _ w481]
          tunnel: [_ _ T21 {"Image Size"=TRUE, "Image Type"=TRUE, "Pixel Value"=TRUE, "ROI Information"=TRUE, "Zoom Factor"=FALSE} ("Image Information Shown:All Elements")] -> w468
          tunnel: [_ _ TRUE ("Zoom Factor")] -> w467
          tunnel: w466 -> [_ _ w478]
          frame Default {
          }
          frame "Stop", "Record" {
            # "Place Window too"
            n300 = invoke class="VI" method="FP.Close"(reference=w477) -> (reference out=w476:refnum<vi>)  [unwired: 2 in, 2 out]
            n301 = invoke class="VI" method="Abort VI"(reference=w476) -> ()  [unwired: 2 in, 3 out]
          }
          frame "Playback" {
            n302 = call "Open Playback Panel.vi"("Offset"=w481, "DB VI Ref"=w482, "Playback in"=w486) -> ("Playback out"=w483:refnum<vi>)  [unwired: 8 in]
            n303 = register-events(w483, w478) -> (reference out=w485:refnum<event-registration>, error out=w484:errorcluster)  [unwired: 2 in]
          }
        }
        n304 = property on="Camera Image" class="ImageControl"("Image Information Shown"=w468, "Image Information Visible"=w467) -> ()  [unwired: 2 in, 2 out]
        n305 = call <vilib>:"WPI_DashboardNT Log FieldName Cache.vi"("Operation"=enum16{"Lookup/Add", "Index", "Clear"}."Clear") -> ()  [unwired: 8 in, 3 out]
      }
      event Panel Close {
        w488 = enum32{"Stop", "Record", "Playback"}."Stop" ("Rec Mode")
        # "Playback window has been closed, abort"
        n306 = event-data() -> ()  [unwired: 1 in, 4 out]
        n307 = local write "Rec Mode"(w488) -> ()
        n308 = global write "WPI_DashboardLogging Global.vi" "Recording"(w488) -> ()
      }
      event Panel Close {
        # "Abort playback window and ourself"
        n309 = event-data() -> ()  [unwired: 1 in, 4 out]
        n310 = invoke class="VI" method="FP.Close"(reference=w492) -> (reference out=w491:refnum<vi>)  [unwired: 2 in, 2 out]
        n311 = invoke class="VI" method="Abort VI"(reference=w491) -> (error out=w490:errorcluster)  [unwired: 2 in, 2 out]
        n312 = invoke class="VI" method="Abort VI"(error in=w490) -> ()  [unwired: 2 in, 3 out]
      }
      event User Event {
        n313 = event-data() -> ("IDs"=w499:cluster{"RPC field ID":u16, "Unique ID":u16}, "String"=w498:string)  [unwired: 1 in]
        n314 = Bundle("IDs"=w499, "String"=w498) -> (w497:T9)  [unwired: 1 in]
        n315 = call <vilib>:"Retrieve RPC Response.vi"("RPC Response"=w497) -> ("Output"=w495:string[][])  [unwired: 10 in]
        n316 = Build Array (concatenate)(w493, w495) -> (w494:string[][])
        n317 = local write "Command Params"(w494) -> ()
        n318 = local write "Cmd Status"("" ("Cmd Status")) -> ()
      }
      event "Tree": Double Click {
        n319 = event-data() -> ("PlatMods"=w503:T24, "Tag"=w502:string)  [unwired: 1 in]
        n320 = Unbundle(w503) -> ("Shift"=w501:bool)  [unwired: 4 out]
        n321 = Not(x=w501) -> (.not. x?=w500:bool)
        n322 = call <vilib>:"NT Update Persistence.vi"("Persistence"=w500, "Name"=w502) -> ()  [unwired: 9 in, 1 out]
      }
    }
  }
  n323 = while {
    tunnel: w64 -> [w506]
    i -> [w509]
    stop <- FALSE stop-if-true
    n324 = Wait (ms)(milliseconds to wait=u32 100) -> ()  [unwired: 1 out]
    n325 = case shown="\"Playback\"" "Rec Mode" {
      tunnel: w509 -> [_ _ w524]
      tunnel: [u32 2829099 ("Base Color") u32 11141120 ("Target Color") w513] -> w505
      frame "Stop", Default {
        # "Reset the color, extra updates don't cost much"
      }
      frame "Record" {
      }
      frame "Playback" {
        # "Playback"
        n326 = Quotient & Remainder(x=w524, y=u32 50 ("milliseconds to wait")) -> (x-y*floor(x/y)=w520:u32)  [unwired: 1 out]
        n327 = Divide(x=w520, y=u32 50 ("milliseconds to wait")) -> (x/y=w517:dbl)
        n328 = Multiply(x=6.283185307179586, y=w517) -> (x*y=w522:dbl)
        n329 = Sine(x=w522) -> (sin(x)=w521:dbl)
        n330 = Absolute Value(x=w521) -> (abs(x)=w514:dbl)
        n331 = call "Interpolate RGB Color.vi"("Proportion"=w514, "Target Color"=u32 30976, "Base Color"=u32 2829099) -> ("Result Color"=w513:u32)  [unwired: 8 in]
      }
    }
    n332 = property class="Pane"(reference=w506, "PaneColor"=w505) -> ()  [unwired: 1 in, 2 out]
  }
  n333 = local write "Dashboard Tab"(T2."Drive" ("Dashboard Tab")) -> ()
  n334 = property on="On/Off" class="Bool (strict)"("Visible"=w34) -> ()  [unwired: 2 in, 2 out]
  n335 = property on="Motor" class="Clust (strict)"("Visible"=w34) -> ()  [unwired: 2 in, 2 out]
  n336 = property on="Progress" class="Clust (strict)"("Visible"=w34) -> ()  [unwired: 2 in, 2 out]
  n337 = property on="Test Ring" class="Ring (strict)"("Visible"=w34) -> ()  [unwired: 2 in, 2 out]
  n338 = property on="Rev/Fwd" class="Clust (strict)"("Visible"=w34) -> ()  [unwired: 2 in, 2 out]
  n339 = local write "Command Selection"(u16 0 ("milliseconds to wait")) -> ()
  n340 = local write "Command Params"(string[][] [] ("Command Params")) -> ()
  n341 = global write "WPI_DashboardLogging Global.vi" "Recording"(w58) -> ()
  n342 = local write "Rec Mode"(w58) -> ()
  n343 = while {
    tunnel: u16 1741 ("timeout ms (25000)") -> [w526]
    stop <- FALSE stop-if-true
    n344 = TCP Create Listener(10:w526) -> (0:w525:errorcluster, 3:w527:refnum<k5>)  [unwired: 4 in, 1 out]
    n345 = case shown="No Error" w525 {
      selector: w525 -> [w529 _]
      tunnel: w527 -> [w530 _]
      frame No Error {
        n346 = while {
          tunnel: w530 -> [w533]
          tunnel: w529 -> [w532]
          stop <- FALSE stop-if-true
          n347 = TCP Wait On Listener(8:w532, 11:w533) -> (0:w534:errorcluster, 4:w535:refnum<k5>)  [unwired: 2 in, 3 out]
          n348 = local write "TCP"(w535) -> ()
          n349 = case shown="No Error" w534 {
            frame No Error {
            }
            frame Error {
              n350 = Wait (ms)(milliseconds to wait=u32 1000) -> ()  [unwired: 1 out]
            }
          }
        }
      }
      frame Error {
        n351 = Wait (ms)(milliseconds to wait=u32 1000) -> ()  [unwired: 1 out]
      }
    }
  }
  n352 = call <vilib>:"NT Write String.vi"("String"="Select Auto", "Name"="Auto Selector") -> ()  [unwired: 9 in, 1 out]
